vi "updateTriggerMode.vi"(8 "error in (no error)":errorcluster, 10 "Pane":refnum<vi>, 11 "ICSettingsViewer in":refnum<class "ICSettingsViewer.lvclass">) -> (0 "error out":errorcluster, 2 "Pane out":refnum<vi>, 3 "ICSettingsViewer out":refnum<class "ICSettingsViewer.lvclass">)   [LabVIEW 2009, in "Views.lvlib" / "Camera.lvlib" / "ICSettingsViewer.lvclass"]
uses:
  ICSettingsViewer.lvclass
  ICSettingsViewer.lvclass/ICSettingsViewer.ctl
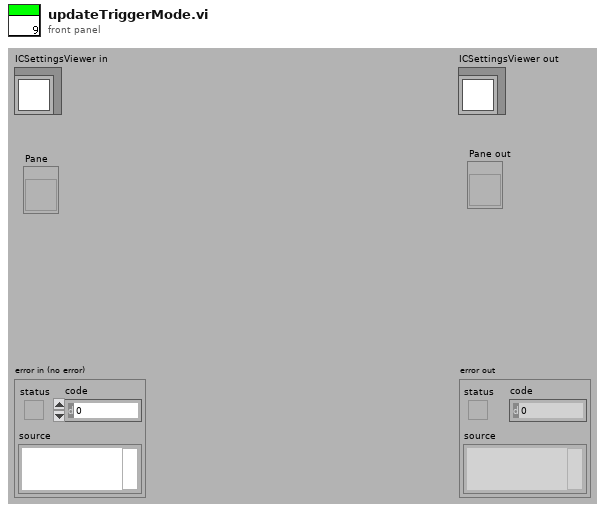
[diagram p1: front panel]
types:
  T1 = enum16{"exposure", "gain", "image_number", "Triggering", "start_trigger"}
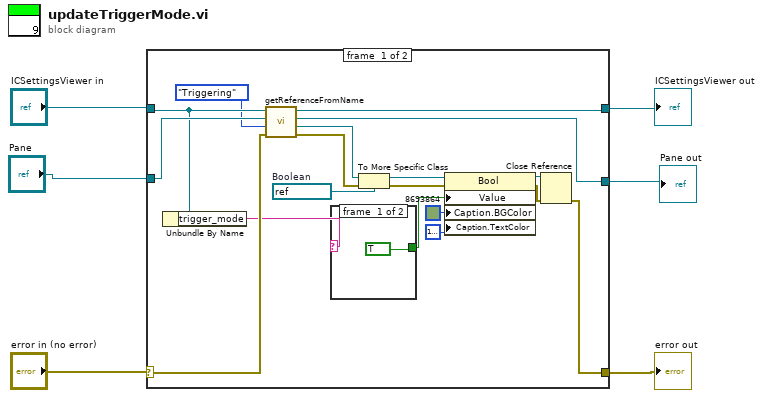
[diagram p0: block diagram]
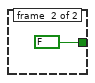
[diagram p2: hidden frame]
diagram:
  n1 = case shown="No Error" "error in (no error)" {
    selector: "error in (no error)" -> [w23 w28]
    tunnel: [w13 w28] -> w3
    tunnel: [w12 w27] -> w1
    tunnel: "ICSettingsViewer in" -> [w16 w27]
    tunnel: "Pane" -> [w24 _]
    tunnel: [w22 _] -> w2
    frame #0 {
      w18 = refnum<vi> refnum  # Boolean
      n2 = Unbundle By Name(w16) -> ("trigger_mode"=w11:string)
      n3 = call "getReferenceFromName.vi"("error in (no error)"=w23, "referenceName"=T1."Triggering", "Pane"=w24, "ICSettingsViewer in"=w16) -> ("error out"=w21:errorcluster, "Ctl Refnum"=w17:refnum<vi>, "Pane out"=w22:refnum<vi>, "ICSettingsViewer out"=w12:refnum<class "ICSettingsViewer.lvclass">)  [unwired: 3 in, 1 out]
      n4 = case shown="\"1\"" w11 {
        tunnel: [TRUE FALSE] -> w10
        frame #0 {
        }
        frame #1 {
        }
      }
      n5 = To More Specific Class(target class=w18, reference=w17, error in=w21) -> (specific class reference=w20:refnum<vi>, error out=w19:errorcluster)
      n6 = property class="Bool"(reference=w20, error in=w19, "Value"=w10, "Caption.BGColor"=u32 8693864, "Caption.TextColor"=u32 16777222) -> (reference out=w15:refnum<vi>, error out=w14:errorcluster)
      n7 = Close Reference(reference=w15, error in (no error)=w14) -> (error out=w13:errorcluster)
    }
    frame #1 {
    }
  }
  "error out" <- w3
  "ICSettingsViewer out" <- w1
  "Pane out" <- w2
